vi "Main_QMH.vi"() -> ()   [LabVIEW 2020]
doc: "Este vi sirve para el control de monturas mecánicas y adquisición de datos de 2 instrumentos físicos.\n\nSolicitante:\nDr. Gabriel Ramos"
uses:
  <instrlib>/ZaberTSeries/Public/Utility/Request.ctl
  <instrlib>/ZaberTSeries/ZaberTSeries.lvlib
  <instrlib>/ZaberTSeries/Public/Utility/Response.ctl
  <instrlib>/Stanford Research 830/Stanford Research 830.lvlib
  <instrlib>/Tektronix TDS 200 1000 2000 Series/Tektronix TDS 200 1000 2000 Series.lvlib
  <instrlib>/Control de MaP/Control de MaP.lvlib
  H:/Mi unidad/Departamento de Ingenieria/Investigadores/Gabriel Ramos/Proyecto Monturas v13/LV Source/Type Definitions/Tipos de montura.ctl
  Type Definitions/Datos Zaber.ctl
  Type Definitions/parametros motores.ctl
  Type Definitions/Datos a Guardar.ctl
  Type Definitions/datos osciloscopio.ctl
  Type Definitions/Asistente de adquisicion Cluster.ctl
  Type Definitions/Program data.ctl
panel:
  in  "Save home":bool
  in  "Avance (mm)":dbl=1.0
  in  "Move backward":bool
  in  "Move forward":bool
  in  "Start acquisition":bool
  in  "Stop Button":bool
  out "Posición Actual (um)":dbl[unit](slide) max=0.05
  out "Datos":dbl[](graph)
  out "Datos actuales":T1
  # "ENA\nDTA"
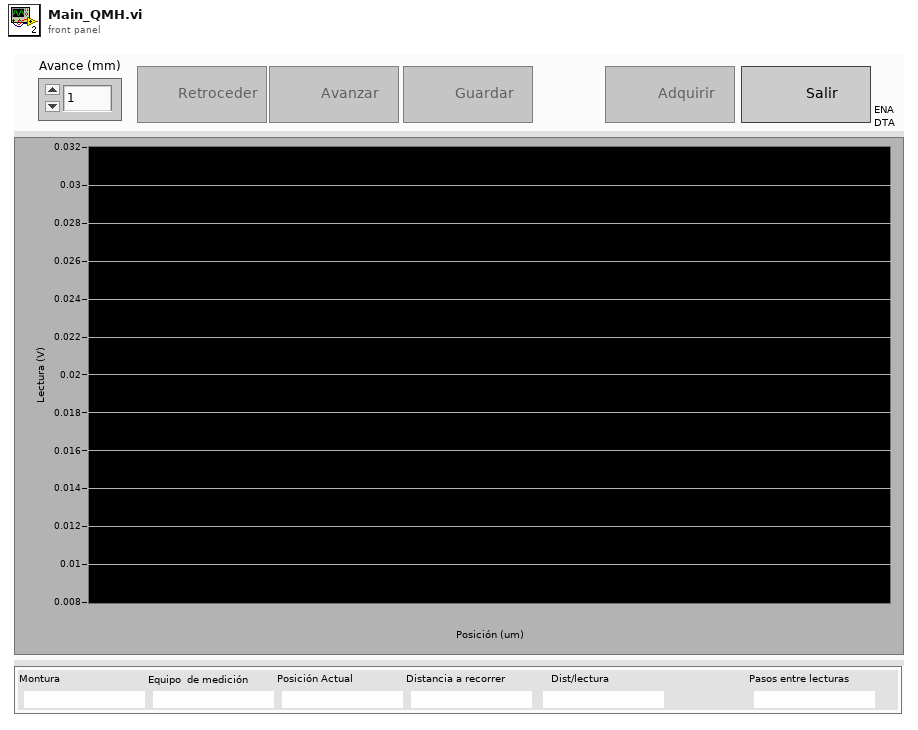
[diagram p1: front panel]
types:
  T1 = cluster{"Montura":string, "Equipo  de medición":string, "Posición Actual":string, "Distancia a recorrer":string, "Dist/lectura":string, "Pasos entre lecturas":string}
  T2 = typedef "Program data.ctl" = cluster{"Acq data":T3, "Meas":dbl[]}
  T3 = typedef "Asistente de adquisicion Cluster.ctl" = cluster{"Equipo a Utilizar":enum16{"SR830 Lock In", "TDS 2012B Osciloscope"}, "Montura":T4, "Datos Zaber":T5, "Datos Bipolar/Unipolar":T6, "Datos Archivo":cluster{"Ruta Archivo":path, "Nombre de Prueba":string}, "Datos actuales":cluster{"Montura":string, "Equipo":string, "Posición Actual":string, "Distancia Total a recorrer":string, "distancia Entre lecturas":string, "Pasos entre lecturas":string}, "Datos a Guardar In":T7, "Datos Osciloscopio":T8, "Datos Lock In":cluster{"Visa Lock in":refnum<visa-resource-name>}}
  T4 = typedef "Tipos de montura.ctl" = enum16{"Zaber T-LSR450B", "Zaber-T-LSR300B", "Zaber-T-LSRxxx", "Motor Bipolar", "Motor Unipolar"}
  T5 = typedef "Datos Zaber.ctl" = cluster{"Sentido de Adquisición":bool, "Comenzar Desde Home?":bool, "Distancia a recorrer (um)":dbl, "Pasos motor":i32, "Distancia entre Lecturas (um)":dbl, "Puerto":refnum<visa-resource-name>}
  T6 = typedef "parametros motores.ctl" = cluster{"Puerto COM":refnum<visa-resource-name>, "Pasos entre Lecturas":u16, "Numero de lecturas":u32, "Sentido del motor":bool}
  T7 = typedef "Datos a Guardar.ctl" = cluster{"Datos Cursor Tektronix":string, "Datos Lokin":string, "Posición Cero":dbl[unit], "Posición Actual":dbl[unit]}
  T8 = typedef "datos osciloscopio.ctl" = cluster{"Sesión Visa Osciloscopio":refnum<visa-resource-name>, "Tipo de Adquisición":enum16{"Voltaje Pico Pico", "Voltaje RMS", "Cursor Tiempo"}, "Canal a Utilizar":enum16{"Canal 1", "Canal 2", "Canal 1 y 2"}, "Parametros de Adquisición":enum16{"Una Muestra", "Promedio"}, "Número Promedio":i32}
  T9 = typedef "ZaberTSeries.lvlib/Response.ctl" = cluster{"Device Number":u8, "Command":u8, "Data":i32}
  T10 = enum8{"Enabled", "Disabled", "Disabled and Grayed Out"}
  T11 = typedef "ZaberTSeries.lvlib/Request.ctl" = cluster{"Device Number":u8, "Command":u8, "Data":i32, "Response Count":i32}
  T12 = cluster{"Montura":string, "Equipo":string, "Posición Actual":string, "Distancia Total a recorrer":string, "distancia Entre lecturas":string, "Pasos entre lecturas":string}
  T13 = typedef "Constante estados proceso adquisición.ctl" = enum16{"Inicializar interfaz", "Inicializar Equipo", "Inicializar Montura", "Leer Pos Actual", "Inicializar Archivo", "Leer Equipo", "guardar Archivo", "Mover Montura", "Corroborar distancias y Stop", "Cerrar Archivo y equipos"}
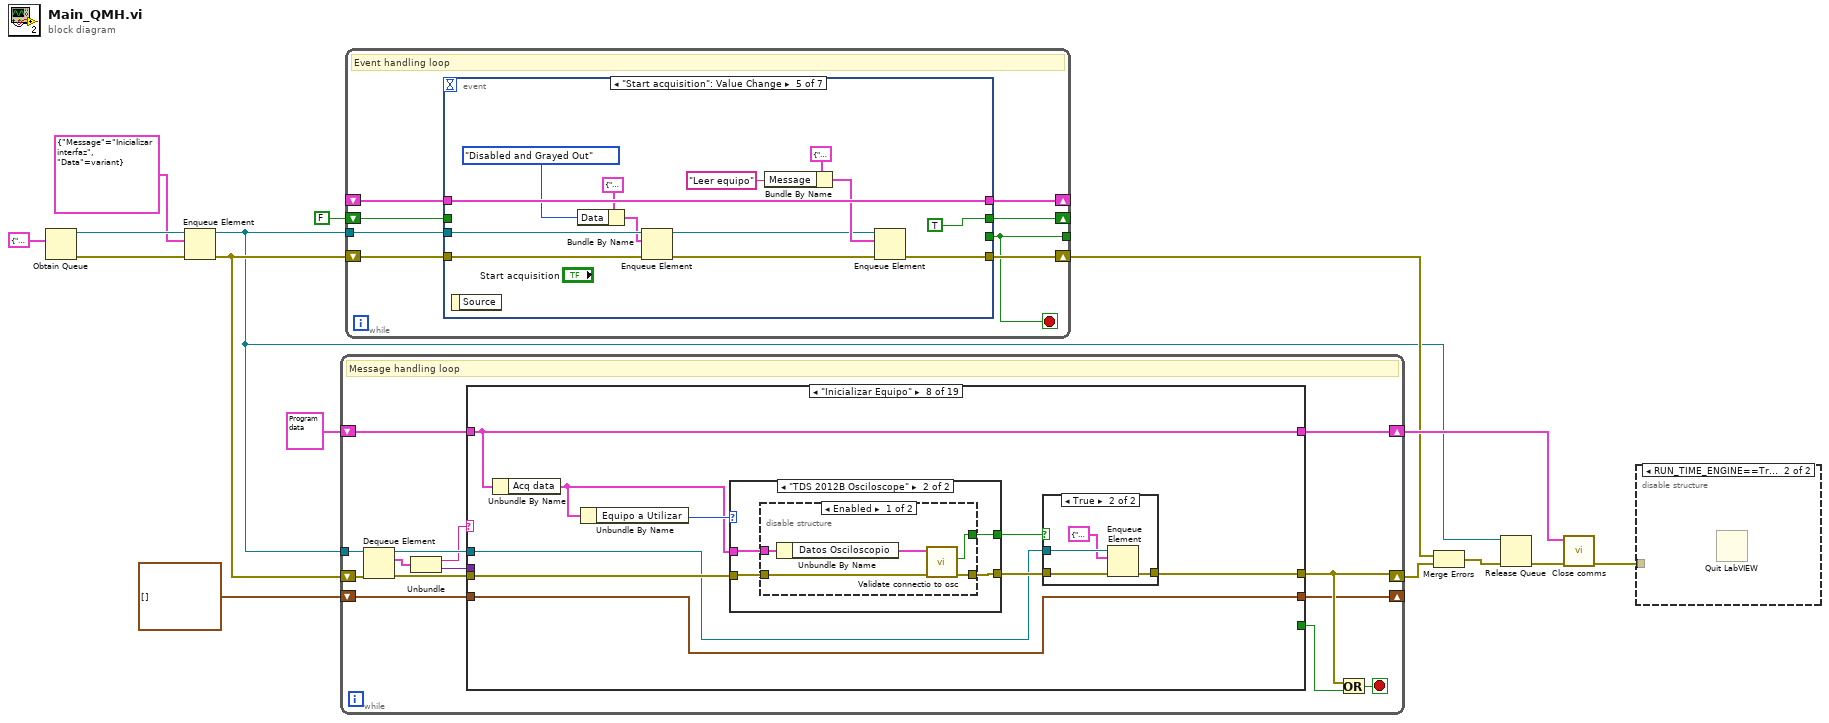
[diagram p0: block diagram]
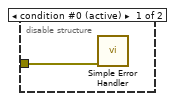
[diagram p2: hidden frame]
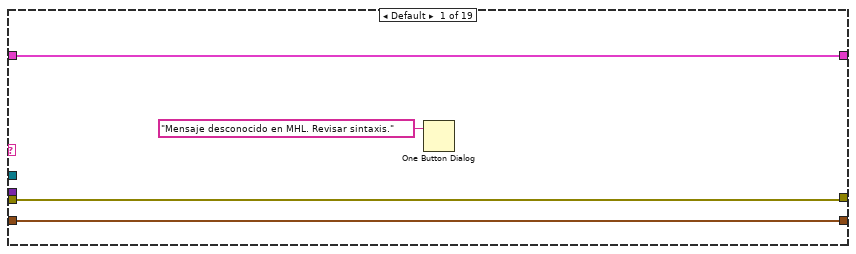
[diagram p3: hidden frame]
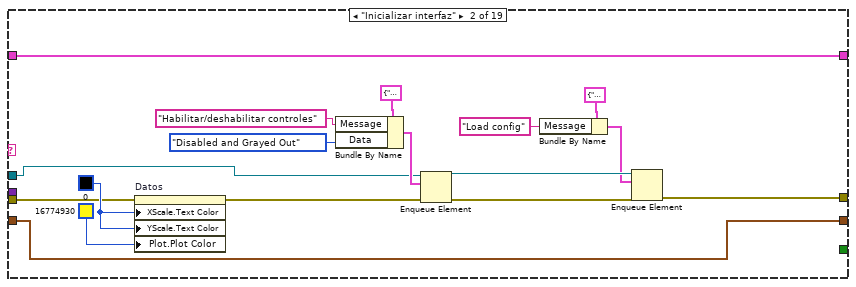
[diagram p4: hidden frame]
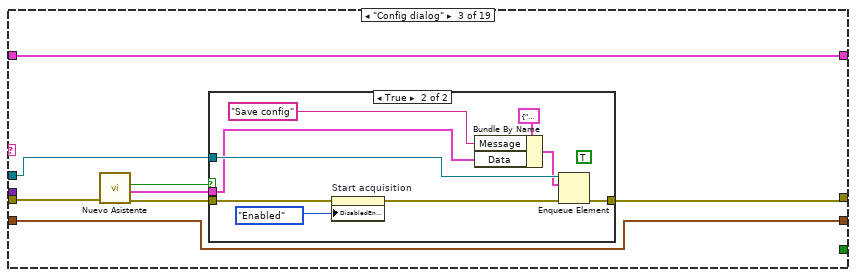
[diagram p5: hidden frame]
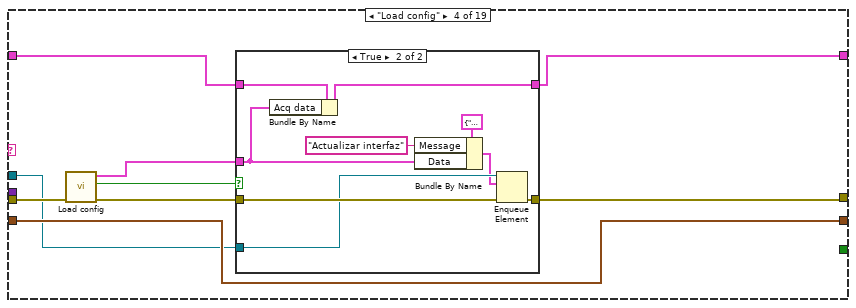
[diagram p7: hidden frame]
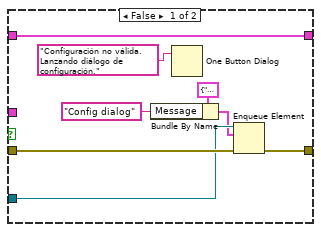
[diagram p8: hidden frame]
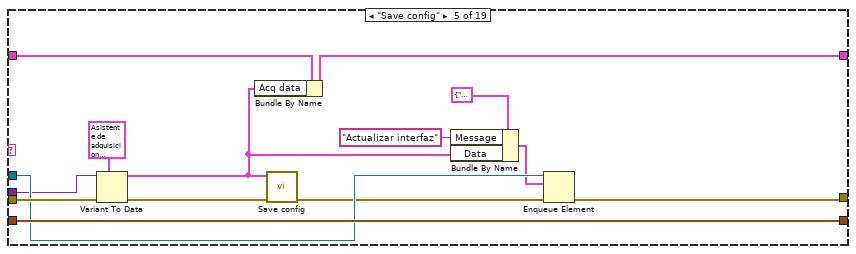
[diagram p9: hidden frame]
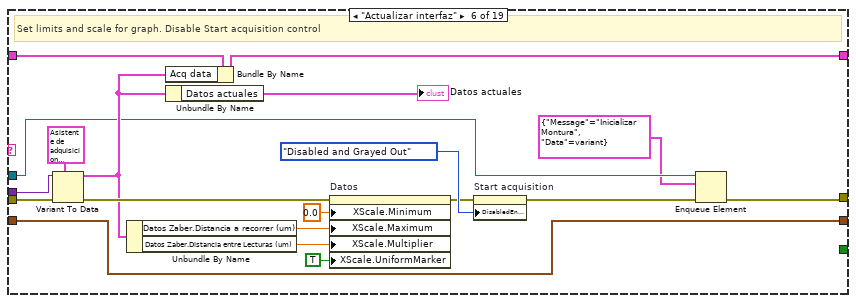
[diagram p10: hidden frame]
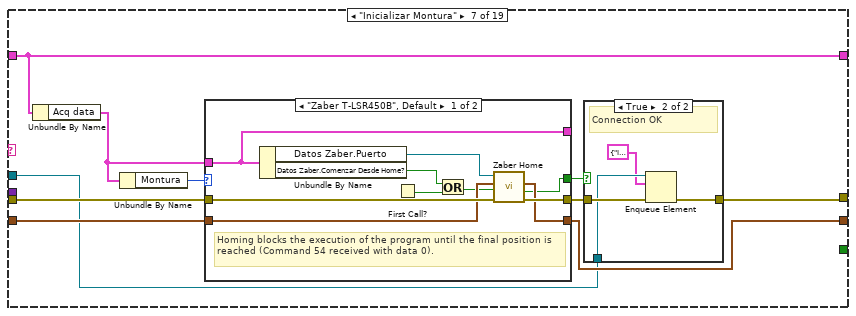
[diagram p11: hidden frame]
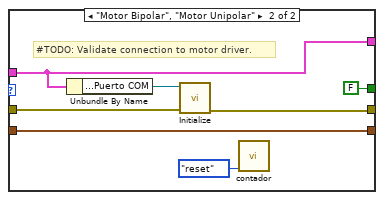
[diagram p13: hidden frame]
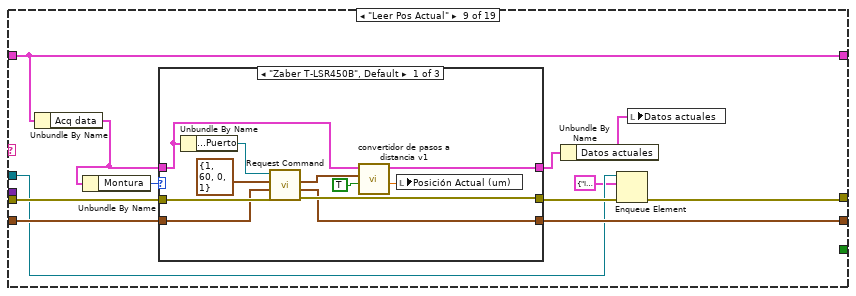
[diagram p17: hidden frame]
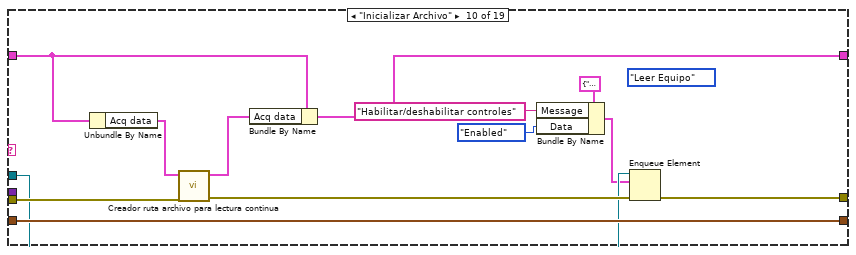
[diagram p20: hidden frame]
diagram:
  n1 = Obtain Queue(element data type=cluster{"Message":string, "Data":variant} {"Message"="", "Data"=variant}) -> (queue out=w9:refnum<queue>, error out=w13:errorcluster)  [unwired: 4 in, 1 out]
  n2 = Enqueue Element(queue=w9, element=cluster{"Message":string, "Data":variant} {"Message"="Inicializar interfaz", "Data"=variant}, error in (no error)=w13) -> (queue out=w2:refnum<queue>, error out=w10:errorcluster)  [unwired: 1 in, 1 out]
  n3 = while {
    tunnel: w2 -> [w29]
    shift-right: [w25] -> w6
    shift-left: w10 -> [w28]
    shift-right: [w20] -> w7
    shift-left: T2 {"Acq data"={"Equipo a Utilizar"=enum."TDS 2012B Osciloscope", "Montura"=enum."Zaber T-LSR450B", "Datos Zaber"={"Sentido de Adquisición"=FALSE, "Comenzar Desde Home?"=FALSE, "Distancia a recorrer (um)"=0.0, "Pasos motor"=0, "Distancia entre Lecturas (um)"=0.0, "Puerto"=""}, "Datos Bipolar/Unipolar"={"Puerto COM"="", "Pasos entre Lecturas"=0, "Numero de lecturas"=0, "Sentido del motor"=TRUE}, "Datos Archivo"={"Ruta Archivo"=path "", "Nombre de Prueba"=""}, "Datos actuales"={"Montura"="", "Equipo"="", "Posición Actual"="", "Distancia Total a recorrer"="", "distancia Entre lecturas"="", "Pasos entre lecturas"=""}, "Datos a Guardar In"={"Datos Cursor Tektronix"="", "Datos Lokin"="", "Posición Cero"=0.0, "Posición Actual"=0.0}, "Datos Osciloscopio"={"Sesión Visa Osciloscopio"="Tektronix_TDS2012C", "Tipo de Adquisición"=enum."Voltaje Pico Pico", "Canal a Utilizar"=enum."Canal 1", "Parametros de Adquisición"=enum."Una Muestra", "Número Promedio"=2}, "Datos Lock In"={"Visa Lock in"="Tektronix_TDS2012C"}}, "Meas"=[]} -> [w21]
    shift-right: [w17] -> _
    shift-left: T9[] [] ("Responses in") -> [w24]
    stop <- w23 stop-if-true
    # "Message handling loop"
    n4 = Dequeue Element(queue=w29, error in (no error)=w28) -> (queue out=w22:refnum<queue>, element=w26:cluster{"Message":string, "Data":variant}, error out=w27:errorcluster)  [unwired: 1 in, 1 out]
    n5 = Unbundle(w26) -> ("Message"=w18:string, "Data"=w19:variant)
    n6 = case shown="\"Inicializar Equipo\"" w18 {
      tunnel: w19 -> [_ _ _ _ w100 w118 _ _ _ _ _ _ _ _ w355 _ _ w413 _]
      tunnel: w27 -> [w33 w47 w54 w76 w108 w126 w136 w167 w195 w225 w238 w268 w287 w320 w357 w367 w381 w417 w421]
      tunnel: [w33 w38 w53 w74 w106 w112 w130 w163 w189 w223 w231 w266 w280 w315 w344 w374 w380 w414 w421] -> w25
      tunnel: w24 -> [w32 w50 w58 w77 w107 w127 w134 w165 w193 w226 w236 w269 w285 w318 w347 w360 w389 w416 w420]
      tunnel: [w32 w50 w58 w77 w107 w127 w133 w165 w192 w226 w236 w269 w284 w317 w346 w358 w389 w416 w420] -> w17
      tunnel: w22 -> [_ w42 w52 w73 w105 w111 w129 w162 w188 w222 w229 w265 w279 w313 _ _ w379 _ _]
      tunnel: w21 -> [w31 w40 w51 w70 w101 w116 w132 w164 w191 w218 w233 w262 w272 w311 w340 w375 w385 w415 w418]
      tunnel: [w31 w40 w51 w69 w99 w115 w132 w164 w191 w219 w228 w262 w270 w309 w338 w375 w385 w415 w418] -> w20
      tunnel: [_ _ _ _ _ _ _ _ _ _ _ _ _ _ _ _ _ _ TRUE] -> w16
      frame Default {
        n7 = One Button Dialog(message="Mensaje desconocido en MHL. Revisar sintaxis.") -> ()  [unwired: 1 in, 1 out]
      }
      frame "Inicializar interfaz" {
        w48 = u32 0 ("X Scale.Marker Colors:Text Color")
        n8 = property on="Datos" class="WFGraph (strict)"(error in=w47, "XScale.Text Color"=w48, "YScale.Text Color"=w48, "Plot.Plot Color"=u32 16774930) -> (error out=w46:errorcluster)  [unwired: 1 in, 1 out]
        n9 = Bundle By Name(cluster=cluster{"Message":string, "Data":variant} {"Message"="Habilitar/deshabilitar controles", "Data"=variant}, "Message"="Habilitar/deshabilitar controles", "Data"=T10."Disabled and Grayed Out" ("Disabled")) -> (w43:cluster{"Message":string, "Data":variant})
        n10 = Enqueue Element(queue=w42, element=w43, error in (no error)=w46) -> (queue out=w35:refnum<queue>, error out=w39:errorcluster)  [unwired: 1 in, 1 out]
        n11 = Bundle By Name(cluster=cluster{"Message":string, "Data":variant} {"Message"="Habilitar/deshabilitar controles", "Data"=variant}, "Message"="Load config") -> (w34:cluster{"Message":string, "Data":variant})
        n12 = Enqueue Element(queue=w35, element=w34, error in (no error)=w39) -> (error out=w38:errorcluster)  [unwired: 1 in, 2 out]
      }
      frame "Config dialog" {
        n13 = call "Nuevo Asistente.vi"("error in (no error)"=w54) -> ("error out"=w56:errorcluster, "Datos de Nueva Adquisición"=w57:T3, "Iniciar Prueba"=w55:bool)  [unwired: 8 in]
        n14 = case shown="True" w55 {
          tunnel: w56 -> [w59 w68]
          tunnel: [w59 w65] -> w53
          tunnel: w57 -> [_ w61]
          tunnel: w52 -> [_ w64]
          frame False {
          }
          frame True {
            (unwired) TRUE
            n15 = property on="Start acquisition" class="Bool"(error in=w68, "DisabledEnum"=T10."Enabled" ("Disabled")) -> (error out=w67:errorcluster)  [unwired: 1 in, 1 out]
            n16 = Bundle By Name(cluster=cluster{"Message":string, "Data":variant} {"Message"="Save config", "Data"=variant}, "Message"="Save config", "Data"=w61) -> (w62:cluster{"Message":string, "Data":variant})
            n17 = Enqueue Element(queue=w64, element=w62, error in (no error)=w67) -> (error out=w65:errorcluster)  [unwired: 1 in, 2 out]
          }
        }
      }
      frame "Load config" {
        n18 = call "Load config.vi"("error in (no error)"=w76) -> ("error out"=w75:errorcluster, "Valid?"=w72:bool, "Datos Adquisición out"=w71:T3)  [unwired: 8 in]
        n19 = case shown="True" w72 {
          tunnel: w75 -> [w85 w94]
          tunnel: [w82 w93] -> w74
          tunnel: w73 -> [w81 w92]
          tunnel: w71 -> [_ w88]
          tunnel: w70 -> [w84 w91]
          tunnel: [w84 w90] -> w69
          frame False {
            n20 = Bundle By Name(cluster=cluster{"Message":string, "Data":variant} {"Message"="Save config", "Data"=variant}, "Message"="Config dialog") -> (w78:cluster{"Message":string, "Data":variant})
            n21 = One Button Dialog(message="Configuración no válida. Lanzando diálogo de configuración.") -> ()  [unwired: 1 in, 1 out]
            n22 = Enqueue Element(queue=w81, element=w78, error in (no error)=w85) -> (error out=w82:errorcluster)  [unwired: 1 in, 2 out]
          }
          frame True {
            n23 = Bundle By Name(cluster=w91, "Acq data"=w88) -> (w90:T2)
            n24 = Bundle By Name(cluster=cluster{"Message":string, "Data":variant} {"Message"="Actualizar interfaz", "Data"=variant}, "Message"="Actualizar interfaz", "Data"=w88) -> (w87:cluster{"Message":string, "Data":variant})
            n25 = Enqueue Element(queue=w92, element=w87, error in (no error)=w94) -> (error out=w93:errorcluster)  [unwired: 1 in, 2 out]
          }
        }
      }
      frame "Save config" {
        n26 = Variant To Data(error in=w108, type=T3 {"Equipo a Utilizar"=enum."TDS 2012B Osciloscope", "Montura"=enum."Zaber T-LSR450B", "Datos Zaber"={"Sentido de Adquisición"=FALSE, "Comenzar Desde Home?"=FALSE, "Distancia a recorrer (um)"=0.0, "Pasos motor"=0, "Distancia entre Lecturas (um)"=0.0, "Puerto"=""}, "Datos Bipolar/Unipolar"={"Puerto COM"="", "Pasos entre Lecturas"=0, "Numero de lecturas"=0, "Sentido del motor"=TRUE}, "Datos Archivo"={"Ruta Archivo"=path "", "Nombre de Prueba"=""}, "Datos actuales"={"Montura"="", "Equipo"="", "Posición Actual"="", "Distancia Total a recorrer"="", "distancia Entre lecturas"="", "Pasos entre lecturas"=""}, "Datos a Guardar In"={"Datos Cursor Tektronix"="", "Datos Lokin"="", "Posición Cero"=0.0, "Posición Actual"=0.0}, "Datos Osciloscopio"={"Sesión Visa Osciloscopio"="Tektronix_TDS2012C", "Tipo de Adquisición"=enum."Voltaje Pico Pico", "Canal a Utilizar"=enum."Canal 1", "Parametros de Adquisición"=enum."Una Muestra", "Número Promedio"=2}, "Datos Lock In"={"Visa Lock in"="Tektronix_TDS2012C"}} ("Acq data"), Variant=w100) -> (data=w96:T3, error out=w103:errorcluster)
        n27 = Bundle By Name(cluster=w101, "Acq data"=w96) -> (w99:T2)
        n28 = call "Save config.vi"("error in (no error)"=w103, "Datos Adquisición"=w96) -> ("error out"=w104:errorcluster)  [unwired: 9 in]
        n29 = Bundle By Name(cluster=cluster{"Message":string, "Data":variant} {"Message"="Actualizar interfaz", "Data"=variant}, "Message"="Actualizar interfaz", "Data"=w96) -> (w95:cluster{"Message":string, "Data":variant})
        n30 = Enqueue Element(queue=w105, element=w95, error in (no error)=w104) -> (error out=w106:errorcluster)  [unwired: 1 in, 2 out]
      }
      frame "Actualizar interfaz" {
        # "Set limits and scale for graph. Disable Start acquisition control"
        n31 = Variant To Data(error in=w126, type=T3 {"Equipo a Utilizar"=enum."TDS 2012B Osciloscope", "Montura"=enum."Zaber T-LSR450B", "Datos Zaber"={"Sentido de Adquisición"=FALSE, "Comenzar Desde Home?"=FALSE, "Distancia a recorrer (um)"=0.0, "Pasos motor"=0, "Distancia entre Lecturas (um)"=0.0, "Puerto"=""}, "Datos Bipolar/Unipolar"={"Puerto COM"="", "Pasos entre Lecturas"=0, "Numero de lecturas"=0, "Sentido del motor"=TRUE}, "Datos Archivo"={"Ruta Archivo"=path "", "Nombre de Prueba"=""}, "Datos actuales"={"Montura"="", "Equipo"="", "Posición Actual"="", "Distancia Total a recorrer"="", "distancia Entre lecturas"="", "Pasos entre lecturas"=""}, "Datos a Guardar In"={"Datos Cursor Tektronix"="", "Datos Lokin"="", "Posición Cero"=0.0, "Posición Actual"=0.0}, "Datos Osciloscopio"={"Sesión Visa Osciloscopio"="Tektronix_TDS2012C", "Tipo de Adquisición"=enum."Voltaje Pico Pico", "Canal a Utilizar"=enum."Canal 1", "Parametros de Adquisición"=enum."Una Muestra", "Número Promedio"=2}, "Datos Lock In"={"Visa Lock in"="Tektronix_TDS2012C"}} ("Datos de Nueva Adquisición"), Variant=w118) -> (data=w114:T3, error out=w119:errorcluster)
        n32 = Unbundle By Name(w114) -> ("Datos Zaber.Distancia a recorrer (um)"=w124:dbl, "Datos Zaber.Distancia entre Lecturas (um)"=w123:dbl)
        n33 = Bundle By Name(cluster=w116, "Acq data"=w114) -> (w115:T2)
        n34 = Unbundle By Name(w114) -> ("Datos actuales"=→"Datos actuales":T12)
        n35 = property on="Datos" class="WFGraph (strict)"(error in=w119, "XScale.Minimum"=0.0 ("X Scale.Range:Minimum"), "XScale.Maximum"=w124, "XScale.Multiplier"=w123, "XScale.UniformMarker"=TRUE ("X Scale.Uniform Marker Spacing?")) -> (error out=w120:errorcluster)  [unwired: 1 in, 1 out]
        n36 = property on="Start acquisition" class="Bool"(error in=w120, "DisabledEnum"=T10."Disabled and Grayed Out" ("Disabled")) -> (error out=w113:errorcluster)  [unwired: 1 in, 1 out]
        n37 = Enqueue Element(queue=w111, element=cluster{"Message":string, "Data":variant} {"Message"="Inicializar Montura", "Data"=variant}, error in (no error)=w113) -> (error out=w112:errorcluster)  [unwired: 1 in, 2 out]
      }
      frame "Inicializar Montura" {
        n38 = Unbundle By Name(w132) -> ("Acq data"=w131:T3)
        n39 = Unbundle By Name(w131) -> ("Montura"=w137:T4)
        n40 = case shown="\"Zaber T-LSR450B\", Default" w137 {
          tunnel: w136 -> [w152 w157]
          tunnel: [w151 w156] -> w135
          tunnel: w131 -> [w148 w155]
          tunnel: w134 -> [w149 w159]
          tunnel: [w147 w159] -> w133
          tunnel: [w148 w155] -> _
          tunnel: [w143 FALSE ("Success?")] -> w128
          frame "Zaber T-LSR450B", Default {
            # "Homing blocks the execution of the program until the final position is reached (Command 54 received with data 0)."
            n41 = Unbundle By Name(w148) -> ("Datos Zaber.Puerto"=w150:refnum<visa-resource-name>, "Datos Zaber.Comenzar Desde Home?"=w145:bool)
            n42 = First Call?() -> (First Call?: T/F=w146:bool)
            n43 = Or(x=w145, y=w146) -> (x .or. y?=w144:bool)
            n44 = call "Zaber Home.vi"("error in (no error)"=w152, "Ir a Home"=w144, "Responses in"=w149, "VISA Refnum in"=w150) -> ("error out"=w151:errorcluster, "Success?"=w143:bool, "Responses out"=w147:T9[])  [unwired: 4 in, 1 out]
          }
          frame "Motor Bipolar", "Motor Unipolar" {
            # "#TODO: Validate connection to motor driver."
            n45 = Unbundle By Name(w155) -> ("Datos Bipolar/Unipolar.Puerto COM"=w158:refnum<visa-resource-name>)
            n46 = call <instrlib>:"Initialize.vi"("error in (no error)"=w157, "Puerto Serial"=w158) -> ("error out"=w156:errorcluster)  [unwired: 8 in, 1 out]
            n47 = call "contador.vi"("Opciones"=enum16{"reset", "mas uno", "lectura"}."reset") -> ()  [unwired: 10 in, 1 out]
          }
        }
        n48 = case shown="True" w128 {
          tunnel: w135 -> [w138 w142]
          tunnel: [w138 w141] -> w130
          tunnel: w129 -> [_ w140]
          frame False {
            # "Connection NOK"
          }
          frame True {
            # "Connection OK"
            n49 = Enqueue Element(queue=w140, element=cluster{"Message":string, "Data":variant} {"Message"="Inicializar Equipo", "Data"=variant}, error in (no error)=w142) -> (error out=w141:errorcluster)  [unwired: 1 in, 2 out]
          }
        }
      }
      frame "Inicializar Equipo" {
        n50 = Unbundle By Name(w164) -> ("Acq data"=w161:T3)
        n51 = Unbundle By Name(w161) -> ("Equipo a Utilizar"=w168:enum16{"SR830 Lock In", "TDS 2012B Osciloscope"})
        n52 = case shown="\"TDS 2012B Osciloscope\"" w168 {
          tunnel: w161 -> [_ w178]
          tunnel: w167 -> [w174 w177]
          tunnel: [w174 w176] -> w166
          tunnel: [_ w175] -> w160
          frame "SR830 Lock In", Default {
          }
          frame "TDS 2012B Osciloscope" {
            n53 = disable-structure shown="Enabled" {
              disable-tunnel: w178 -> [w183 _]
              disable-tunnel: w177 -> [w181 w184]
              disable-tunnel: [w180 w184] -> w176
              disable-tunnel: [w179 _] -> w175
              frame Enabled {
                n54 = Unbundle By Name(w183) -> ("Datos Osciloscopio"=w182:T8)
                n55 = call "Validate connectio to osc.vi"("error in (no error)"=w181, "Datos Osciloscopio"=w182) -> ("error out"=w180:errorcluster, "Success?"=w179:bool)  [unwired: 8 in]
              }
              frame Disabled {
              }
            }
          }
        }
        n56 = case shown="True" w160 {
          tunnel: w166 -> [w169 w173]
          tunnel: [w169 w172] -> w163
          tunnel: w162 -> [_ w171]
          frame False {
          }
          frame True {
            n57 = Enqueue Element(queue=w171, element=cluster{"Message":string, "Data":variant} {"Message"="Leer Pos Actual", "Data"=variant}, error in (no error)=w173) -> (error out=w172:errorcluster)  [unwired: 1 in, 2 out]
          }
        }
      }
      frame "Leer Pos Actual" {
        n58 = Unbundle By Name(w191) -> ("Acq data"=w190:T3)
        n59 = Unbundle By Name(w190) -> ("Montura"=w196:T4)
        n60 = case shown="\"Zaber T-LSR450B\", Default" w196 {
          tunnel: w195 -> [w207 w210 w213]
          tunnel: [w206 w210 w213] -> w194
          tunnel: w190 -> [w198 w208 w211]
          tunnel: w193 -> [w205 w209 w212]
          tunnel: [w204 w209 w212] -> w192
          tunnel: [w197 w208 w211] -> w186
          frame "Zaber T-LSR450B", Default {
            n61 = Unbundle By Name(w198) -> ("Datos Zaber.Puerto"=w202:refnum<visa-resource-name>)
            n62 = call <instrlib>:"Request Command.vi"("error in (no error)"=w207, "Responses in"=w205, "Request"=T11 {"Device Number"=1, "Command"=60, "Data"=0, "Response Count"=1}, "VISA resource name"=w202) -> ("error out"=w206:errorcluster, "Responses out"=w204:T9[], "First Response"=w200:T9)  [unwired: 4 in, 1 out]
            n63 = call "convertidor de pasos a distancia v1.vi"("Set 0 vitual"=TRUE ("Inicializar"), "Respuesta Zaber"=w200, "Datos adquisición Input"=w198) -> ("Respuesta conversión zaber"=w203:dbl[unit], "Datos adquisición Out"=w197:T3)  [unwired: 6 in, 1 out]
            n64 = local write "Posición Actual (um)"(w203) -> ()
          }
          frame "Motor Bipolar" {
          }
          frame "Motor Unipolar" {
          }
        }
        n65 = Unbundle By Name(w186) -> ("Datos actuales"=w185:T12)
        n66 = Enqueue Element(queue=w188, element=cluster{"Message":string, "Data":variant} {"Message"="Inicializar Archivo", "Data"=variant}, error in (no error)=w194) -> (error out=w189:errorcluster)  [unwired: 1 in, 2 out]
        n67 = local write "Datos actuales"(w185) -> ()
      }
      frame "Inicializar Archivo" {
        (unwired) Constante_estados_proceso_adquisición."Leer Equipo" ("f")
        n68 = Unbundle By Name(w218) -> ("Acq data"=w217:T3)
        n69 = call "Creador ruta archivo para lectura continua.vi"("error in (no error)"=w225, "Datos de Nueva Adquisición In"=w217) -> ("error out"=w224:errorcluster, "Datos de Nueva Adquisición out"=w220:T3)  [unwired: 4 in]
        n70 = Bundle By Name(cluster=w218, "Acq data"=w220) -> (w219:T2)
        n71 = Bundle By Name(cluster=cluster{"Message":string, "Data":variant} {"Message"="Habilitar/deshabilitar controles", "Data"=variant} ("element"), "Message"="Habilitar/deshabilitar controles", "Data"=T10."Enabled" ("Disabled")) -> (w216:cluster{"Message":string, "Data":variant})
        n72 = Enqueue Element(queue=w222, element=w216, error in (no error)=w224) -> (error out=w223:errorcluster)  [unwired: 1 in, 2 out]
      }
      frame "Leer equipo" {
        n73 = Unbundle By Name(w233) -> ("Meas"=w234:dbl[], "Acq data"=w232:T3)
        n74 = Unbundle By Name(w232) -> ("Equipo a Utilizar"=w239:enum16{"SR830 Lock In", "TDS 2012B Osciloscope"})
        n75 = case shown="\"TDS 2012B Osciloscope\"" w239 {
          tunnel: w232 -> [w242 w256]
          tunnel: w238 -> [w244 w260]
          tunnel: [w243 w259] -> w237
          tunnel: [w240 w257] -> w235
          tunnel: [w241 w255] -> _
          frame "TDS 2012B Osciloscope" {
            n76 = disable-structure shown="Enabled" {
              disable-tunnel: w244 -> [w251 w252]
              disable-tunnel: [w250 w252] -> w243
              disable-tunnel: w242 -> [w249 w253]
              disable-tunnel: [w248 w253] -> w241
              disable-tunnel: [w246 _] -> w240
              frame Enabled {
                n77 = Unbundle By Name(w249) -> ("Datos Osciloscopio"=w247:T8)
                n78 = call "Tektronix cursor Read.vi"("error in (no error)"=w251, "Datos Osciloscopio"=w247) -> ("error out"=w250:errorcluster, "Dato"=w245:string, "CH1"=w246:dbl)  [unwired: 7 in]
                n79 = Bundle By Name(cluster=w249, "Datos a Guardar In.Datos Cursor Tektronix"=w245) -> (w248:T3)
              }
              frame Disabled {
              }
            }
          }
          frame "SR830 Lock In" {
            w258 = u16 1 items=["X"=1, "Y"=2, "R"=3, "Theta"=4, "Channel 1"=5, "Channel 2"=6, "Aux In 1"=7, "Aux In 2"=8, "Aux In 3"=9, "Aux In 4"=10] ("Parameter (1: X)")
            n80 = Unbundle By Name(w256) -> ("Datos Lock In.Visa Lock in"=w261:refnum<visa-resource-name>)
            n81 = call "sr830 dsp lock in.vi"("error in (no error)"=w260, "Parameter (1: X)"=w258, "VISA resource name"=w261) -> ("error out"=w259:errorcluster, "Datos Lokin String"=w254:string, "Medición"=w257:dbl)  [unwired: 6 in]
            n82 = Bundle By Name(cluster=w256, "Datos a Guardar In.Datos Lokin"=w254) -> (w255:T3)
          }
        }
        n83 = Build Array (concatenate)(w234, w235) -> (w227:dbl[])
        "Datos" <- w227
        n84 = Bundle By Name(cluster=w233, "Meas"=w227) -> (w228:T2)
        n85 = Enqueue Element(queue=w229, element=cluster{"Message":string, "Data":variant} {"Message"="guardar Archivo", "Data"=variant}, error in (no error)=w237) -> (error out=w231:errorcluster)  [unwired: 1 in, 2 out]
      }
      frame "guardar Archivo" {
        n86 = Unbundle By Name(w262) -> ("Acq data"=w263:T3)
        n87 = call "Guardar datos.vi"("error in"=w268, "Datos de Nueva Adquisición"=w263) -> ("error out"=w267:errorcluster)  [unwired: 8 in, 1 out]
        n88 = Enqueue Element(queue=w265, element=cluster{"Message":string, "Data":variant} {"Message"="Corroborar distancias y Stop", "Data"=variant}, error in (no error)=w267) -> (error out=w266:errorcluster)  [unwired: 1 in, 2 out]
      }
      frame "Corroborar distancias y Stop" {
        # "#TODO: final position = current position + travel"
        n89 = Unbundle By Name(w272) -> ("Acq data"=w281:T3)
        n90 = Unbundle By Name(w281) -> ("Montura"=w288:T4)
        n91 = case shown="\"Zaber T-LSR450B\"" w288 {
          tunnel: w287 -> [w299 w308]
          tunnel: [w298 w308] -> w286
          tunnel: w285 -> [w300 w307]
          tunnel: [w297 w307] -> w284
          tunnel: w281 -> [w289 w301]
          tunnel: [w296 w302] -> w283
          tunnel: [w290 w301] -> w271
          tunnel: [w295 w306] -> w282
          frame "Zaber T-LSR450B" {
            # "Query for position and update indicator."
            n92 = Unbundle By Name(w289) -> ("Datos Zaber.Puerto"=w294:refnum<visa-resource-name>)
            n93 = call <instrlib>:"Request Command.vi"("error in (no error)"=w299, "Responses in"=w300, "Request"=T11 {"Device Number"=1, "Command"=60, "Data"=0, "Response Count"=1}, "VISA resource name"=w294) -> ("error out"=w298:errorcluster, "Responses out"=w297:T9[], "First Response"=w292:T9)  [unwired: 4 in, 1 out]
            n94 = call "convertidor de pasos a distancia v1.vi"("Set 0 vitual"=FALSE ("Inicializar"), "Respuesta Zaber"=w292, "Datos adquisición Input"=w289) -> ("Respuesta conversión zaber"=w295:dbl[unit], "Datos adquisición Out"=w290:T3, "Seguir Moviendo"=w296:bool)  [unwired: 6 in]
          }
          frame "Motor Bipolar", Default {
            n95 = Unbundle By Name(w301) -> ("Datos Bipolar/Unipolar.Numero de lecturas"=w303:u32)
            n96 = call "contador.vi"("Opciones"=enum16{"reset", "mas uno", "lectura"}."lectura") -> ("Contador"=w304:i32)  [unwired: 10 in]
            n97 = node(w304) -> (w306:dbl[unit])
            n98 = Less Or Equal?(x=w304, y=w303) -> (x <= y?=w302:bool)
          }
        }
        "Posición Actual (um)" <- w282
        n99 = Select(t="Mover Montura", s=w283, f="Cerrar Archivo y equipos") -> (s? t:f=w274:string)
        n100 = Unbundle By Name(w271) -> ("Datos actuales"=w273:T12)
        n101 = Bundle By Name(cluster=w272, "Acq data"=w271) -> (w270:T2)
        n102 = Bundle By Name(cluster=cluster{"Message":string, "Data":variant} {"Message"="", "Data"=variant} ("element"), "Message"=w274) -> (w277:cluster{"Message":string, "Data":variant})
        n103 = Enqueue Element(queue=w279, element=w277, error in (no error)=w286) -> (error out=w280:errorcluster)  [unwired: 1 in, 2 out]
        n104 = local write "Datos actuales"(w273) -> ()
      }
      frame "Mover Montura" {
        n105 = Unbundle By Name(w311) -> ("Acq data"=w316:T3)
        n106 = Unbundle By Name(w316) -> ("Montura"=w321:T4)
        n107 = case shown="\"Zaber T-LSR450B\", Default" w321 {
          tunnel: w320 -> [w332 w336]
          tunnel: [w331 w335] -> w319
          tunnel: w316 -> [w322 w333]
          tunnel: w318 -> [w329 w337]
          tunnel: [w328 w337] -> w317
          tunnel: [w324 w333] -> w310
          frame "Zaber T-LSR450B", Default {
            # "Moving blocks the execution of the program until the final position is reached (Command 54 received with data 0)."
            # "Send a relative position according to the number of steps calculated as resolution."
            n108 = Unbundle By Name(w322) -> ("Datos Zaber.Puerto"=w330:refnum<visa-resource-name>, "Datos Zaber"=w323:T5)
            n109 = call "Extractor pasos para montura zaber.vi"("Datos Zaber"=w323) -> ("to Zaber"=w327:T11)  [unwired: 10 in]
            n110 = call <instrlib>:"Request Command.vi"("error in (no error)"=w332, "Responses in"=w329, "Request"=w327, "VISA resource name"=w330) -> ("error out"=w331:errorcluster, "Responses out"=w328:T9[], "First Response"=w326:T9)  [unwired: 4 in, 1 out]
            n111 = call "convertidor de pasos a distancia v1.vi"("Respuesta Zaber"=w326, "Datos adquisición Input"=w322) -> ("Respuesta conversión zaber"=w325:dbl[unit], "Datos adquisición Out"=w324:T3)  [unwired: 7 in, 1 out]
            n112 = local write "Posición Actual (um)"(w325) -> ()
          }
          frame "Motor Bipolar", "Motor Unipolar" {
            n113 = call "Motion control Custom motor.vi"("error in (no error)"=w336, "Datos de Nueva Adquisición"=w333) -> ("error out"=w335:errorcluster)  [unwired: 9 in]
            n114 = call "contador.vi"("Opciones"=enum16{"reset", "mas uno", "lectura"}."mas uno") -> ()  [unwired: 10 in, 1 out]
          }
        }
        n115 = Unbundle By Name(w310) -> ("Datos actuales"=w312:T12)
        n116 = Bundle By Name(cluster=w311, "Acq data"=w310) -> (w309:T2)
        n117 = local write "Datos actuales"(w312) -> ()
        n118 = Enqueue Element(queue=w313, element=cluster{"Message":string, "Data":variant} {"Message"="Leer Equipo", "Data"=variant}, error in (no error)=w319) -> (error out=w315:errorcluster)  [unwired: 1 in, 2 out]
      }
      frame "Jog" {
        w342 = FALSE  # Set 0 vitual
        # "#TODO: add logic for steppers."
        n119 = Variant To Data(error in=w357, type=FALSE, Variant=w355) -> (data=w352:bool, error out=w345:errorcluster)
        n120 = Unbundle By Name(w340) -> ("Acq data"=w343:T3)
        n121 = call "Get motor command.vi"("Direction (F = Backward)"=w352, "Avance"="Avance (mm)") -> ("Datos Zaber"=w356:T5)  [unwired: 9 in]
        n122 = Unbundle By Name(w343) -> ("Datos Zaber.Puerto"=w348:refnum<visa-resource-name>)
        n123 = call "Extractor pasos para montura zaber.vi"("Datos Zaber"=w356) -> ("to Zaber"=w349:T11)  [unwired: 10 in]
        n124 = call <instrlib>:"Request Command.vi"("error in (no error)"=w345, "Responses in"=w347, "Request"=w349, "VISA resource name"=w348) -> ("error out"=w344:errorcluster, "Responses out"=w346:T9[], "First Response"=w351:T9)  [unwired: 4 in, 1 out]
        n125 = call "convertidor de pasos a distancia v1.vi"("Set 0 vitual"=w342, "Respuesta Zaber"=w351, "Datos adquisición Input"=w343) -> ("Respuesta conversión zaber"=w350:dbl[unit], "Datos adquisición Out"=w339:T3)  [unwired: 6 in, 1 out]
        n126 = local write "Posición Actual (um)"(w350) -> ()
        n127 = Unbundle By Name(w339) -> ("Datos actuales"=w341:T12)
        n128 = Bundle By Name(cluster=w340, "Acq data"=w339) -> (w338:T2)
        n129 = local write "Datos actuales"(w341) -> ()
      }
      frame "Guardar Home" {
        # "Return current position."
        # "Command 47 sets the passed position as Home offset."
        n130 = Unbundle By Name(w375) -> ("Acq data"=w363:T3)
        n131 = Unbundle By Name(w363) -> ("Datos Zaber.Puerto"=w366:refnum<visa-resource-name>)
        n132 = Bundle By Name(cluster=T11 {"Device Number"=1, "Command"=0, "Data"=0, "Response Count"=1} ("Request"), "Command"=u8 60) -> (w365:T11)
        n133 = call <instrlib>:"Request Command.vi"("error in (no error)"=w367, "Responses in"=w360, "Request"=w365, "VISA resource name"=w366) -> ("error out"=w368:errorcluster, "Responses out"=w359:T9[], "First Response"=w362:T9, "VISA resource name out"=w364:refnum<visa-resource-name>)  [unwired: 4 in]
        n134 = Unbundle By Name(w362) -> ("Data"=w361:i32)
        n135 = Bundle By Name(cluster=T11 {"Device Number"=1, "Command"=0, "Data"=0, "Response Count"=1} ("Request"), "Command"=u8 47, "Data"=w361) -> (w372:T11)
        n136 = call <instrlib>:"Write Command.vi"("error in (no error)"=w368, "Responses in"=w359, "Request"=w372, "VISA resource name"=w364) -> ("error out"=w374:errorcluster, "Responses out"=w358:T9[])  [unwired: 5 in, 1 out]
      }
      frame "Cerrar Archivo y equipos" {
        n137 = Unbundle By Name(w385) -> ("Acq data"=w384:T3)
        n138 = Unbundle By Name(w384) -> ("Equipo a Utilizar"=w382:enum16{"SR830 Lock In", "TDS 2012B Osciloscope"}, "Montura"=w383:T4)
        n139 = case shown="\"Zaber T-LSR450B\"" w383 {
          tunnel: w389 -> [w402 _]
          tunnel: w381 -> [w401 w404]
          tunnel: [w400 w403] -> w388
          tunnel: w384 -> [w399 w405]
          frame "Zaber T-LSR450B" {
            n140 = Unbundle By Name(w399) -> ("Datos Zaber.Puerto"=w398:refnum<visa-resource-name>)
            n141 = call <instrlib>:"Close.vi"("error in (no error)"=w401, "Responses in"=w402, "VISA resource name"=w398) -> ("error out"=w400:errorcluster)  [unwired: 7 in, 1 out]
          }
          frame "Motor Unipolar", Default {
            n142 = disable-structure shown="Enabled" {
              disable-tunnel: w405 -> [w409 _]
              disable-tunnel: w404 -> [w407 w410]
              disable-tunnel: [w406 w410] -> w403
              frame Enabled {
                n143 = Unbundle By Name(w409) -> ("Datos Bipolar/Unipolar.Puerto COM"=w408:refnum<visa-resource-name>)
                n144 = call <instrlib>:"Close.vi"("error in (no error)"=w407, "VISA resource name"=w408) -> ("error out"=w406:errorcluster)  [unwired: 9 in]
              }
              frame Disabled {
              }
            }
          }
        }
        n145 = case shown="\"TDS 2012B Osciloscope\"" w382 {
          tunnel: w384 -> [w393 w397]
          tunnel: w388 -> [w391 w395]
          tunnel: [w390 w394] -> w386
          frame "SR830 Lock In", Default {
            n146 = Unbundle By Name(w393) -> ("Datos Lock In.Visa Lock in"=w392:refnum<visa-resource-name>)
            n147 = call <instrlib>:"Close.vi"("error in (no error)"=w391, "VISA resource name"=w392) -> ("error out"=w390:errorcluster)  [unwired: 9 in]
          }
          frame "TDS 2012B Osciloscope" {
            n148 = Unbundle By Name(w397) -> ("Datos Lock In.Visa Lock in"=w396:refnum<visa-resource-name>)
            n149 = call <instrlib>:"Close.vi"("error in (no error)"=w395, "VISA resource name"=w396) -> ("error out"=w394:errorcluster)  [unwired: 9 in]
          }
        }
        n150 = call <vilib>:"Clear Errors.vi"("error in (no error)"=w386) -> ("error out"=w387:errorcluster)  [unwired: 5 in, 1 out]
        n151 = Bundle By Name(cluster=cluster{"Message":string, "Data":variant} {"Message"="Habilitar/deshabilitar controles", "Data"=variant}, "Data"=T10."Enabled" ("Disabled")) -> (w376:cluster{"Message":string, "Data":variant})
        n152 = Enqueue Element(queue=w379, element=w376, error in (no error)=w387) -> (error out=w380:errorcluster)  [unwired: 1 in, 2 out]
      }
      frame "Habilitar/deshabilitar controles" {
        n153 = Variant To Data(error in=w417, type=T10."Enabled" ("Disabled"), Variant=w413) -> (data=w411:T10, error out=w414:errorcluster)
        n154 = property on="Start acquisition" class="Bool"("DisabledEnum"=w411) -> ()  [unwired: 2 in, 2 out]
        n155 = property on="Move backward" class="Bool"("DisabledEnum"=w411) -> ()  [unwired: 2 in, 2 out]
        n156 = property on="Move forward" class="Bool"("DisabledEnum"=w411) -> ()  [unwired: 2 in, 2 out]
        n157 = property on="Save home" class="Bool"("DisabledEnum"=w411) -> ()  [unwired: 2 in, 2 out]
      }
      frame "Exit" {
      }
    }
    n158 = Or(x=w25, y=w16) -> (x .or. y?=w23:bool)
  }
  n159 = while {
    tunnel: w2 -> [w429]
    tunnel: [w422] -> _
    shift-right: [w427] -> w3
    shift-left: w10 -> [w428]
    shift-right: [w426] -> _
    shift-left: _ -> [w425]
    shift-right: [w423] -> _
    shift-left: FALSE -> [w424]
    stop <- w422 stop-if-true
    # "Event handling loop"
    n160 = event shown="[4] \"Start acquisition\": Value Change" {
      selector: _ -> [_ _ _ _ _ _ _]
      dyn-events: _ -> [_ _ _ _ _ _ _]
      timeout: _ -> [_ _ _ _ _ _ _]
      tunnel: w429 -> [_ w441 w516 w526 w536 w554 w560]
      tunnel: w428 -> [w432 w439 w518 w528 w538 w556 w562]
      tunnel: [w432 w440 w517 w527 w543 w555 w561] -> w427
      tunnel: [_ w435 TRUE ("NewVal") TRUE ("NewVal") _ _ _] -> w422
      tunnel: [w431 w437 w519 w529 w540 w558 w564] -> w426
      tunnel: w425 -> [w431 w436 w519 w529 w540 w558 w564]
      tunnel: w424 -> [w430 w434 w520 w530 _ w557 w563]
      tunnel: [w430 w433 w520 w530 TRUE w557 w563] -> w423
      event Timeout {
        n161 = event-data() -> ()  [unwired: 1 in, 2 out]
      }
      event Menu Selection (User) {
        n162 = event-data() -> ("ItemTag"=w438:string)  [unwired: 1 in]
        n163 = case shown="\"Salir\"" w438 {
          tunnel: w441 -> [w446 w462 w502 w507]
          tunnel: [w447 w463 w502 w507] -> _
          tunnel: [w448 w469 w500 w508] -> w440
          tunnel: w439 -> [w449 w464 w500 w511]
          tunnel: [w443 w466 w503 w512] -> w437
          tunnel: w436 -> [w445 w465 w503 w512]
          tunnel: [_ _ _ TRUE] -> w435
          tunnel: w434 -> [w444 w467 w501 w509]
          tunnel: [w442 w468 w501 w509] -> w433
          frame "Repetir Adquisición", Default {
            n164 = case shown="True" w444 {
              selector: w444 -> [w450 w457]
              tunnel: w449 -> [w452 w461]
              tunnel: [w452 w460] -> w448
              tunnel: [w453 w459] -> w447
              tunnel: w446 -> [w453 w458]
              tunnel: w445 -> [w451 w455]
              tunnel: [w451 w455] -> w443
              tunnel: [w450 w457] -> w442
              frame False {
              }
              frame True {
                n165 = Bundle By Name(cluster=cluster{"Message":string, "Data":variant} {"Message"="Inicializar montura", "Data"=variant} ("element"), "Data"=w455) -> (w454:cluster{"Message":string, "Data":variant})
                n166 = Enqueue Element(queue=w458, element=w454, error in (no error)=w461) -> (queue out=w459:refnum<queue>, error out=w460:errorcluster)  [unwired: 1 in, 1 out]
              }
            }
          }
          frame "Nueva adquisición" {
            n167 = disable-structure shown="Enabled" {
              disable-tunnel: [w479 w499] -> w469
              disable-tunnel: [w476 _] -> w468
              disable-tunnel: w467 -> [w475 _]
              disable-tunnel: [w473 w497] -> w466
              disable-tunnel: w465 -> [w472 w497]
              disable-tunnel: w464 -> [w471 w498]
              disable-tunnel: w462 -> [w470 w493]
              disable-tunnel: [_ w493] -> w463
              frame Disabled {
                n168 = call "Nuevo Asistente.vi"("error in (no error)"=w471) -> ("error out"=w477:errorcluster, "Datos de Nueva Adquisición"=w474:T3, "Iniciar Prueba"=w478:bool)  [unwired: 8 in]
                n169 = case shown="True" w478 {
                  tunnel: [w480 TRUE] -> w476
                  tunnel: w477 -> [w482 w491]
                  tunnel: [w482 w488] -> w479
                  tunnel: w474 -> [_ w484]
                  tunnel: [w481 w484] -> w473
                  tunnel: w472 -> [w481 _]
                  tunnel: w475 -> [w480 _]
                  tunnel: w470 -> [_ w487]
                  frame False {
                  }
                  frame True {
                    n170 = property on="Start acquisition" class="Bool"(error in=w491, "DisabledEnum"=T10."Enabled" ("Disabled")) -> (error out=w490:errorcluster)  [unwired: 1 in, 1 out]
                    n171 = Bundle By Name(cluster=cluster{"Message":string, "Data":variant} {"Message"="Save config", "Data"=variant}, "Message"="Save data", "Data"=w484) -> (w485:cluster{"Message":string, "Data":variant})
                    n172 = Enqueue Element(queue=w487, element=w485, error in (no error)=w490) -> (error out=w488:errorcluster)  [unwired: 1 in, 2 out]
                  }
                }
              }
              frame Enabled {
                n173 = Bundle By Name(cluster=cluster{"Message":string, "Data":variant} {"Message"="Save config", "Data"=variant}, "Message"="Config dialog") -> (w494:cluster{"Message":string, "Data":variant})
                n174 = Enqueue Element(queue=w493, element=w494, error in (no error)=w498) -> (error out=w499:errorcluster)  [unwired: 1 in, 2 out]
              }
            }
          }
          frame "Osciloscopio en Tiempo Real" {
            n175 = call "Tektronix TDS 200 1000 2000 Series Acquire Continuous Waveform.vi"() -> ()  [unwired: 1 in]
          }
          frame "Salir" {
            n176 = Bundle By Name(cluster=cluster{"Message":string, "Data":variant} {"Message"="Habilitar/deshabilitar controles", "Data"=variant}, "Message"="Exit") -> (w504:cluster{"Message":string, "Data":variant})
            n177 = Enqueue Element(queue=w507, element=w504, error in (no error)=w511) -> (error out=w508:errorcluster)  [unwired: 1 in, 2 out]
          }
        }
      }
      event "Stop Button": Value Change {
        n178 = event-data() -> ()  [unwired: 1 in, 1 out]
        n179 = Bundle By Name(cluster=cluster{"Message":string, "Data":variant} {"Message"="Habilitar/deshabilitar controles", "Data"=variant}, "Message"="Exit") -> (w513:cluster{"Message":string, "Data":variant})
        n180 = Enqueue Element(queue=w516, element=w513, error in (no error)=w518) -> (error out=w517:errorcluster)  [unwired: 1 in, 2 out]
      }
      event Panel Close? {
        n181 = event-data() -> ()  [unwired: 1 in, 1 out]
        n182 = Bundle By Name(cluster=cluster{"Message":string, "Data":variant} {"Message"="Habilitar/deshabilitar controles", "Data"=variant}, "Message"="Exit") -> (w523:cluster{"Message":string, "Data":variant})
        n183 = Enqueue Element(queue=w526, element=w523, error in (no error)=w528) -> (error out=w527:errorcluster)  [unwired: 1 in, 2 out]
        n184 = event-data("Discard?"=TRUE) -> ()  [unwired: 1 in, 1 out]
      }
      event "Start acquisition": Value Change {
        n185 = event-data() -> ()  [unwired: 1 in, 1 out]
        n186 = Bundle By Name(cluster=cluster{"Message":string, "Data":variant} {"Message"="Habilitar/deshabilitar controles", "Data"=variant}, "Data"=T10."Disabled and Grayed Out" ("Disabled")) -> (w533:cluster{"Message":string, "Data":variant})
        n187 = Enqueue Element(queue=w536, element=w533, error in (no error)=w538) -> (queue out=w532:refnum<queue>, error out=w537:errorcluster)  [unwired: 1 in, 1 out]
        n188 = Bundle By Name(cluster=cluster{"Message":string, "Data":variant} {"Message"="", "Data"=variant} ("element"), "Message"="Leer equipo") -> (w539:cluster{"Message":string, "Data":variant})
        n189 = Enqueue Element(queue=w532, element=w539, error in (no error)=w537) -> (error out=w543:errorcluster)  [unwired: 1 in, 2 out]
      }
      event "Move forward", "Move backward": Value Change {
        n190 = event-data() -> ("CtlRef"=w550:refnum<vi>)  [unwired: 1 in]
        n191 = control-ref of="Move forward"() -> (w549:refnum<vi>)
        n192 = Equal?(x=w549, y=w550) -> (x = y?=w548:bool)
        n193 = Select(t=TRUE, s=w548, f=FALSE) -> (s? t:f=w545:bool)
        n194 = Bundle By Name(cluster=cluster{"Message":string, "Data":variant} {"Message"="", "Data"=variant}, "Message"="Jog", "Data"=w545) -> (w551:cluster{"Message":string, "Data":variant})
        n195 = Enqueue Element(queue=w554, element=w551, error in (no error)=w556) -> (error out=w555:errorcluster)  [unwired: 1 in, 2 out]
      }
      event "Save home": Value Change {
        n196 = event-data() -> ()  [unwired: 1 in, 1 out]
        n197 = Enqueue Element(queue=w560, element=cluster{"Message":string, "Data":variant} {"Message"="Guardar Home", "Data"=variant}, error in (no error)=w562) -> (error out=w561:errorcluster)  [unwired: 1 in, 2 out]
      }
    }
  }
  n198 = Merge Errors(w3, w6) -> (w4:errorcluster)
  n199 = Release Queue(queue=w2, error in (no error)=w4) -> (error out=w5:errorcluster)  [unwired: 1 in, 2 out]
  n200 = call "Close comms.vi"("error in (no error)"=w5, "Program data"=w7) -> ("error out"=w1:errorcluster)  [unwired: 9 in]
  n201 = disable-structure shown="RUN_TIME_ENGINE==True" {
    disable-tunnel: w1 -> [w565 _]
    frame condition #0 (active) {
      n202 = call <vilib>:"Simple Error Handler.vi"("error in (no error)"=w565) -> ()  [unwired: 4 in, 5 out]
    }
    frame condition #1 {
      n203 = Quit LabVIEW() -> ()  [unwired: 1 in]
    }
  }
